vi "logging_data_string_to_log_string.vi"(3 "Force binary format (F)":bool, 4 "Raw string to log":string) -> (1 "Result log string":string)   [LabVIEW 2014, in "rszvl_rsidr_core.lvlib"]
uses:
  rszvl_rsidr_core.lvlib
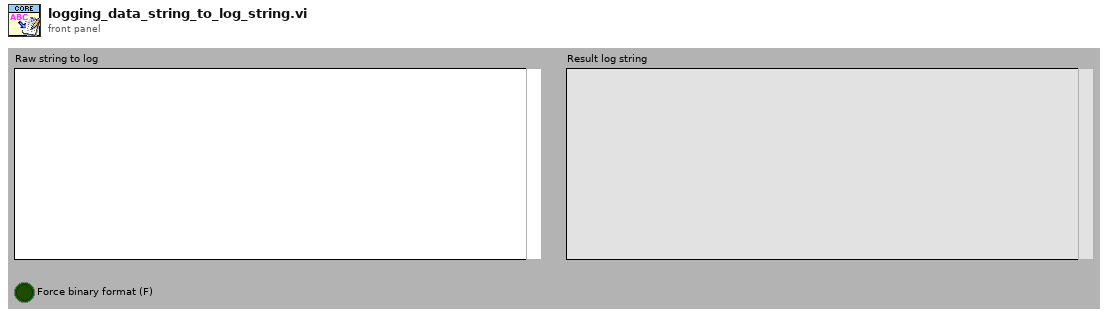
[diagram p1: front panel]
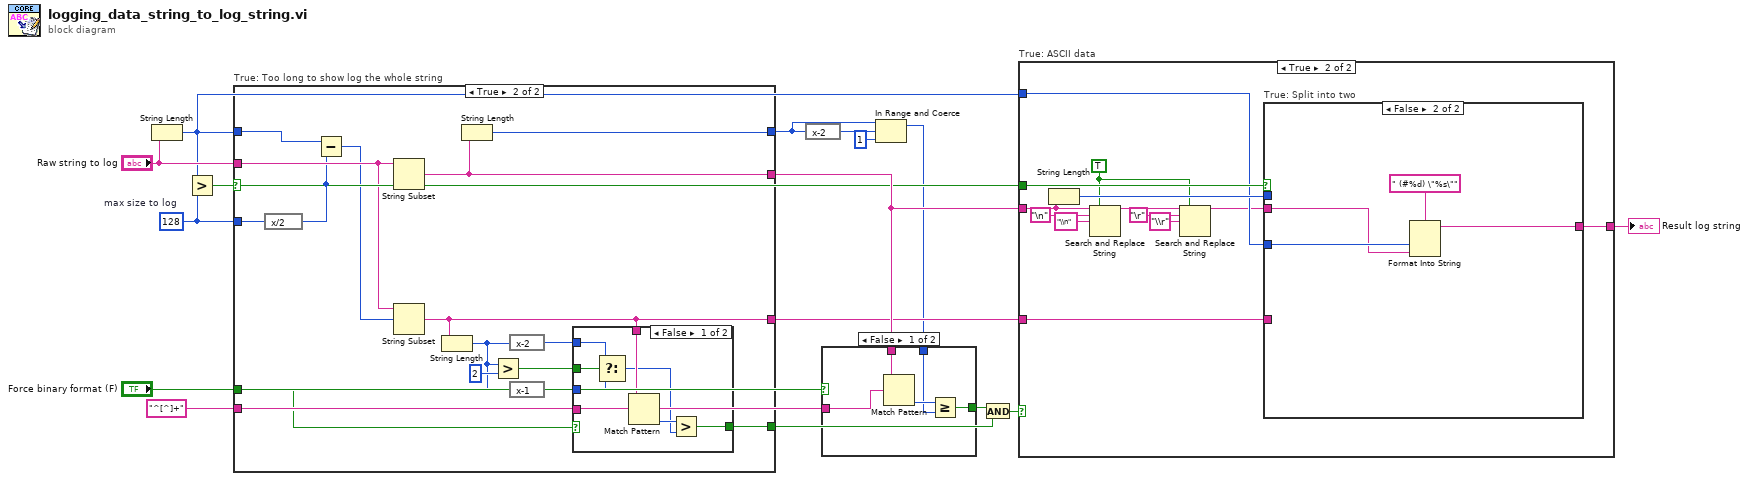
[diagram p0: block diagram]
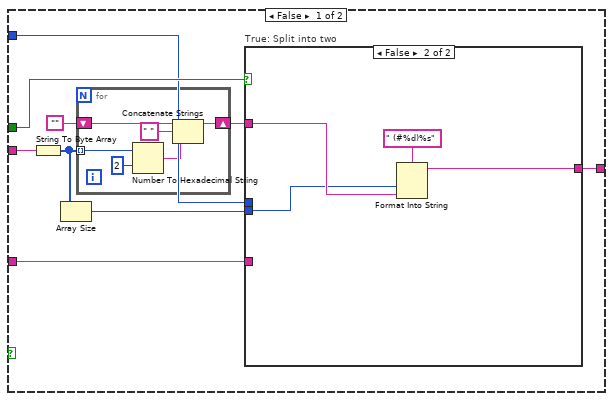
[diagram p3: hidden frame]
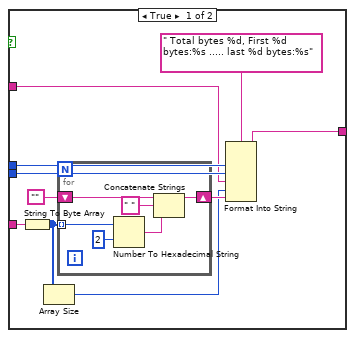
[diagram p4: hidden frame]
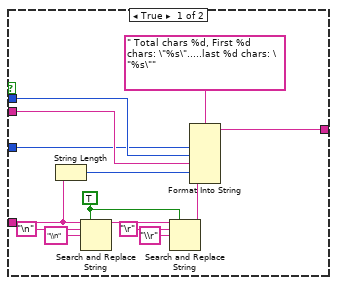
[diagram p5: hidden frame]
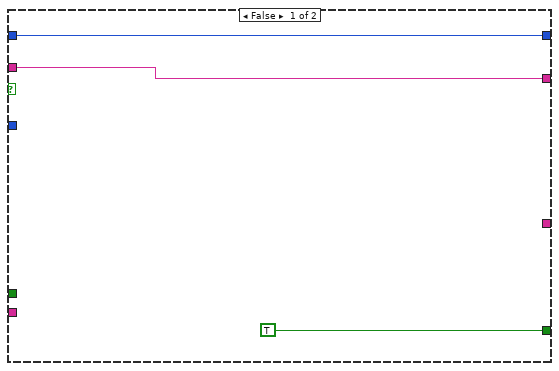
[diagram p6: hidden frame]
diagram:
  w13 = "^[^]+" ("regular expression")
  w15 = 128  # max size to log
  n1 = String Length(string="Raw string to log") -> (length=w9:i32)
  n2 = Greater?(x=w9, y=w15) -> (0:w11:bool)
  n3 = case "True: Too long to show log the whole string" shown="True" w11 {
    tunnel: "Raw string to log" -> [w19 w34]
    tunnel: w15 -> [_ w35]
    tunnel: w9 -> [w18 w33]
    tunnel: [w19 w30] -> w14
    tunnel: [w18 w31] -> w1
    tunnel: [_ w24] -> w12
    tunnel: w13 -> [_ w23]
    tunnel: [TRUE w22] -> w7
    tunnel: "Force binary format (F)" -> [_ w20]
    frame False {
    }
    frame True {
      n4 = expression code="x/2"(w35) -> (w21:i32)
      n5 = Subtract(x=w33, y=w21) -> (x-y=w32:i32)
      n6 = String Subset(string=w34, length (rest)=w21) -> (substring=w30:string)  [unwired: 1 in]
      n7 = String Subset(string=w34, offset (0)=w32) -> (substring=w24:string)  [unwired: 1 in]
      n8 = String Length(string=w24) -> (length=w25:i32)
      n9 = String Length(string=w30) -> (length=w31:i32)
      n10 = Greater?(x=w25, y=2) -> (0:w28:bool)
      n11 = expression code="x-2"(w25) -> (w27:i32)
      n12 = expression code="x-1"(w25) -> (w26:i32)
      n13 = case shown="False" w20 {
        tunnel: w28 -> [w43 _]
        tunnel: w27 -> [w42 _]
        tunnel: w26 -> [w41 _]
        tunnel: w24 -> [w40 _]
        tunnel: w23 -> [w39 _]
        tunnel: [w36 _] -> w22
        frame False {
          n14 = Select(t=w42, s=w43, f=w41) -> (s? t:f=w37:i32)
          n15 = Match Pattern(string=w40, regular expression=w39) -> (offset past match=w38:i32)  [unwired: 1 in, 3 out]
          n16 = Greater?(x=w38, y=w37) -> (0:w36:bool)
        }
        frame True {
        }
      }
    }
  }
  n17 = expression code="x-2"(w1) -> (w4:i32)
  n18 = In Range and Coerce(upper limit=w1, x=w4, lower limit=1) -> (coerced(x)=w3:i32)  [unwired: 1 out]
  n19 = case shown="False" "Force binary format (F)" {
    tunnel: w3 -> [w47 _]
    tunnel: w14 -> [w46 _]
    tunnel: w13 -> [w45 _]
    tunnel: [w44 _] -> w6
    frame False {
      n20 = Match Pattern(string=w46, regular expression=w45) -> (offset past match=w48:i32)  [unwired: 1 in, 3 out]
      n21 = Greater Or Equal?(x=w48, y=w47) -> (x >= y?=w44:bool)
    }
    frame True {
    }
  }
  n22 = And(x=w6, y=w7) -> (x .and. y?=w5:bool)
  n23 = case "True: ASCII data" shown="True" w5 {
    tunnel: w14 -> [w56 w92]
    tunnel: w12 -> [w55 w93]
    tunnel: w11 -> [w57 w94]
    tunnel: [w50 w90] -> w10
    tunnel: w9 -> [w49 w89]
    frame False {
      n24 = String To Byte Array(string=w56) -> (unsigned byte array=w51:u8[])
      n25 = Array Size(array=w51) -> (size(s)=w52:i32)
      n26 = for {
        tunnel: w51 -> [w63] mode=indexing
        shift-right: [w61] -> w53
        shift-left: "" ("Empty String Constant") -> [w60]
        n27 = Number To Hexadecimal String(1:i16 2 ("width (-)"), 2:w63) -> (0:w58:string)
        n28 = Concatenate Strings(w60, " " ("string"), w58) -> (w61:string)
      }
      n29 = case "True: Split into two" shown="False" w57 {
        tunnel: w55 -> [w72 _]
        tunnel: w53 -> [w66 w82]
        tunnel: w52 -> [w69 w81]
        tunnel: [w68 w80] -> w50
        tunnel: w49 -> [w67 _]
        frame True {
          n30 = String To Byte Array(string=w72) -> (unsigned byte array=w65:u8[])
          n31 = Array Size(array=w65) -> (size(s)=w64:i32)
          n32 = for {
            tunnel: w65 -> [w79] mode=indexing
            shift-right: [w77] -> w70
            shift-left: "" ("Empty String Constant") -> [w76]
            n33 = Number To Hexadecimal String(1:i16 2 ("width (-)"), 2:w79) -> (0:w74:string)
            n34 = Concatenate Strings(w76, " " ("string"), w74) -> (w77:string)
          }
          n35 = Format Into String(format string=" Total bytes %d, First %d bytes:%s ..... last %d bytes:%s", w67, w69, w66, w64, w70) -> (resulting string=w68:string)  [unwired: 2 in, 1 out]
        }
        frame False {
          n36 = Format Into String(format string=" (#%d)%s", w81, w82) -> (resulting string=w80:string)  [unwired: 2 in, 1 out]
        }
      }
    }
    frame True {
      w85 = TRUE ("replace all? (F)")
      n37 = String Length(string=w92) -> (length=w91:i32)
      n38 = Search and Replace String(replace all?=w85, input string=w92, search string="\n" ("Line Feed Constant"), replace string="\\n" ("replace string (\"\")")) -> (result string=w86:string)  [unwired: 4 in, 3 out]
      n39 = Search and Replace String(replace all?=w85, input string=w86, search string="\r" ("Carriage Return Constant"), replace string="\\r" ("replace string (\"\")")) -> (result string=w84:string)  [unwired: 4 in, 3 out]
      n40 = case "True: Split into two" shown="False" w94 {
        tunnel: w93 -> [w106 _]
        tunnel: w84 -> [w104 w111]
        tunnel: w91 -> [w107 w112]
        tunnel: [w105 w113] -> w90
        tunnel: w89 -> [w102 _]
        frame True {
          w99 = TRUE ("replace all? (F)")
          n41 = String Length(string=w106) -> (length=w103:i32)
          n42 = Search and Replace String(replace all?=w99, input string=w106, search string="\n" ("Line Feed Constant"), replace string="\\n" ("replace string (\"\")")) -> (result string=w101:string)  [unwired: 4 in, 3 out]
          n43 = Search and Replace String(replace all?=w99, input string=w101, search string="\r" ("Carriage Return Constant"), replace string="\\r" ("replace string (\"\")")) -> (result string=w100:string)  [unwired: 4 in, 3 out]
          n44 = Format Into String(format string=" Total chars %d, First %d chars: \"%s\".....last %d chars: \"%s\"", w102, w107, w104, w103, w100) -> (resulting string=w105:string)  [unwired: 2 in, 1 out]
        }
        frame False {
          n45 = Format Into String(format string=" (#%d) \"%s\"", w112, w111) -> (resulting string=w113:string)  [unwired: 2 in, 1 out]
        }
      }
    }
  }
  "Result log string" <- w10
